vi "(SubVI)_Average.vi"(10 "Index Array":dbl[](array[numeric]), 11 "Data Array":dbl[](array[numeric])) -> (3 "Average":dbl)   [LabVIEW 2012]
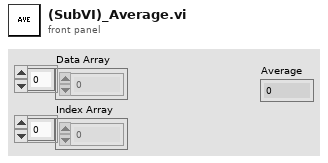
[diagram p1: front panel]
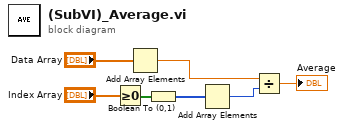
[diagram p0: block diagram]
diagram:
  n1 = Greater Or Equal To 0?(x="Index Array") -> (x >= 0?=w7:bool[])
  n2 = Add Array Elements(numeric array="Data Array") -> (sum=w6:dbl)
  n3 = Boolean To (0,1)(Boolean=w7) -> (0, 1=w5:i16[])
  n4 = Add Array Elements(numeric array=w5) -> (sum=w1:i16)
  n5 = Divide(x=w6, y=w1) -> (x/y=→"Average":dbl)
